vi "Configure Custom Measurement.vi"(6 "Measurement Parameters (S11)":string="S11", 7 "Measurement Type (Standard)":string="Standard", 8 "error in (no error)":errorcluster, 9 "Measurement Name (CH1_S11_1)":string="CH1_S11_1", 10 "Channel (1)":i32=1, 11 "VISA resource name":refnum<visa-resource-name>) -> (0 "error out":errorcluster, 3 "VISA resource name out":refnum<visa-resource-name>)   [LabVIEW 2018, in "Keysight PNA Series.lvlib"]
doc: "Creates a custom measurement."
uses:
  Keysight PNA Series.lvlib
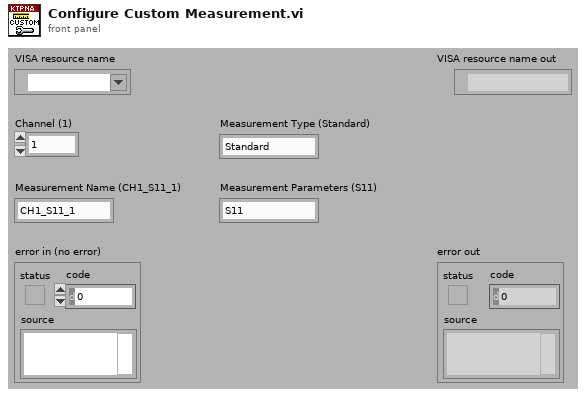
[diagram p1: front panel]
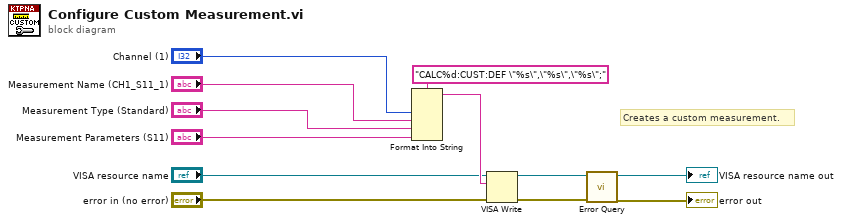
[diagram p0: block diagram]
diagram:
  # "Creates a custom measurement."
  n1 = Format Into String(format string="CALC%d:CUST:DEF \"%s\",\"%s\",\"%s\";", "Channel (1)", "Measurement Name (CH1_S11_1)", "Measurement Type (Standard)", "Measurement Parameters (S11)") -> (resulting string=w7:string)  [unwired: 2 in, 1 out]
  n2 = VISA Write(VISA resource name="VISA resource name", write buffer=w7, error in (no error)="error in (no error)") -> (VISA resource name out=w4:refnum<visa-resource-name>, error out=w3:errorcluster)  [unwired: 1 out]
  n3 = call "Error Query.vi"("error in (no error)"=w3, "VISA resource name"=w4) -> ("error out"=→"error out":errorcluster, "VISA resource name out"=→"VISA resource name out":refnum<visa-resource-name>)  [unwired: 6 in, 2 out]
